vi "Message to the user.vi"() -> ()   [LabVIEW 2015]
panel:
  out "String":string="1234567890abcdefghijklmnopqrstuvwxyz!\"£$%^&*()_+-="
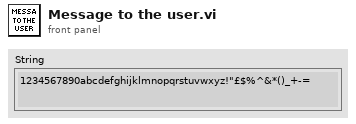
[diagram p1: front panel]
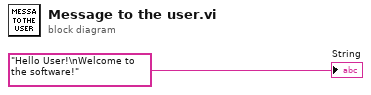
[diagram p0: block diagram]
diagram:
  "String" <- "Hello User!\nWelcome to the software!"
